vi "Read SnP File.vi"   [LabVIEW 2023, in "NI_HFNetworkAnalysis.lvlib"]
doc: "Reads S-parameters from the specified SnP file, assuming Touchstone File Format specifications.\n\n<b>Known limitation</b>\nSupport for S-parameter data only."
uses:
  NI_HFNetworkAnalysis.lvlib
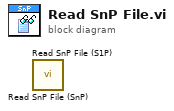
[diagram p0: block diagram]
diagram:
  n1 = call "Read SnP File (SnP).vi"() -> ()  [unwired: 12 in, 4 out]
  n2 = call "Read SnP File (S1P).vi"() -> ()  [unwired: 12 in, 4 out]
